vi "Run.vi"(8 "error in (no error)":errorcluster, 11 "SiemensDigitalEnergyMeter in":refnum<class "SiemensDigitalEnergyMeter.lvclass">) -> (0 "error out":errorcluster, 1 "DataValid":bool, 2 "clSensorData":T1, 3 "SiemensDigitalEnergyMeter out":refnum<class "SiemensDigitalEnergyMeter.lvclass">)   [LabVIEW 2018, in "SensorPlugins.lvlib" / "SiemensDigitalEnergyMeter.lvclass"]
doc: "This VI retrieves measurements from the Siemens Digital Energy Meter."
uses:
  SiemensDigitalEnergyMeter.lvclass
  SensorShared/clSensorData.ctl
  SensorShared/SiemensDEMMeasurements.ctl
  <vilib>/NI/Modbus Library/API/Master/Modbus Master.lvclass
  SensorShared/SensorShared.lvlib
panel:
  out "Execution Time (ms)":u32
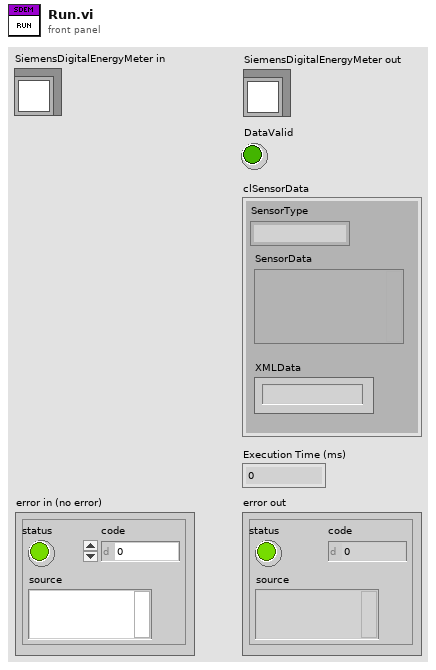
[diagram p1: front panel]
types:
  T1 = typedef "SensorShared.lvlib/clSensorData.ctl" = cluster{"SensorType":string, "SensorData":variant, "XMLData":string}
  T2 = typedef "SensorPlugins.lvlib/SiemensDigitalEnergyMeter.lvclass/CommunicationControls.ctl" = refnum<class "Modbus Master.lvclass">[]
  T3 = typedef "SensorPlugins.lvlib/SiemensDigitalEnergyMeter.lvclass/SiemensDigitalEnergyMeterControls.ctl" = cluster{"Measurement(s)":u16[], "Configuration Commands":string, "Use Measurement Commands Text Box?":bool, "Measurement Commands":string, "Connected?":bool, "Serial Number":string, "IP Address":string, "Port (502)":u16, "Unit ID":u8, "Serial Type":enum16{"RTU", "ASCII"}, "Using TCP?":bool, "VISA Resource Name":string}[]
  T4 = typedef "SensorPlugins.lvlib/SiemensDigitalEnergyMeter.lvclass/MeasurementControls.ctl" = cluster{"Measurement RefreshTime (ms)":u32, "Measurement Name":string}
  T5 = typedef "SensorShared.lvlib/SiemensDEMMeasurements.ctl" = cluster{"Array of Waveforms":waveform(dbl)[], "Array of Strings ":string[]}
  T6 = cluster{"Measurement(s)":u16[], "Configuration Commands":string, "Use Measurement Commands Text Box?":bool, "Measurement Commands":string, "Connected?":bool, "Serial Number":string, "IP Address":string, "Port (502)":u16, "Unit ID":u8, "Serial Type":enum16{"RTU", "ASCII"}, "Using TCP?":bool, "VISA Resource Name":string}
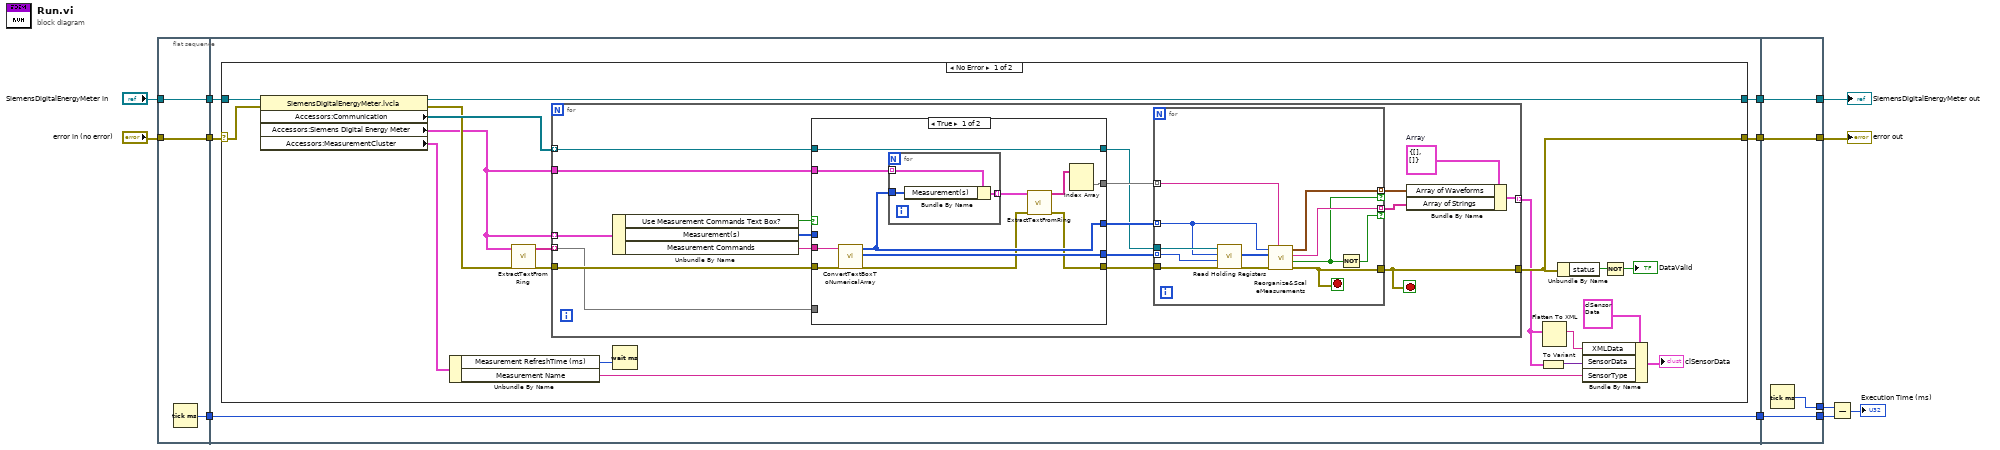
[diagram p0: block diagram]
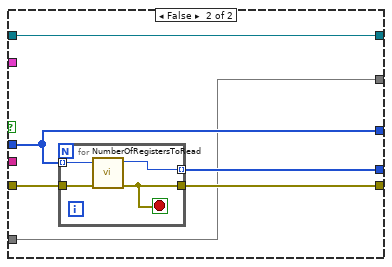
[diagram p2: hidden frame]
diagram:
  n1 = flat-sequence {
    tunnel: "SiemensDigitalEnergyMeter in" -> [w15]
    tunnel: "error in (no error)" -> [w16]
    tunnel: [w16] -> w9
    tunnel: [w15] -> w8
    tunnel: [w14] -> w7
    tunnel: w9 -> [w21]
    tunnel: w8 -> [w20]
    tunnel: [w19] -> w6
    tunnel: [w18] -> w5
    tunnel: w7 -> [w17]
    tunnel: [w17] -> w4
    tunnel: [w99] -> w10
    tunnel: [w100] -> w11
    tunnel: w4 -> [w97]
    tunnel: w5 -> [w99]
    tunnel: w6 -> [w100]
    tunnel: [w98] -> w2
    tunnel: [w97] -> w1
    frame #0 {
      n2 = Tick Count (ms)() -> (millisecond timer value=w14:u32)
    }
    frame #1 {
      n3 = case shown="No Error" w21 {
        selector: w21 -> [w39 w96]
        tunnel: w20 -> [w40 w95]
        tunnel: [w27 w96] -> w18
        tunnel: [w38 w95] -> w19
        frame No Error {
          n4 = property class="SiemensDigitalEnergyMeter.lvcla"(reference=w40, error in=w39) -> (reference out=w38:refnum<class "SiemensDigitalEnergyMeter.lvclass">, error out=w33:errorcluster, "Accessors:Communication"=w37:T2, "Accessors:Siemens Digital Energy Meter"=w30:T3, "Accessors:MeasurementCluster"=w26:T4)
          n5 = Unbundle By Name(w26) -> ("Measurement RefreshTime (ms)"=w25:u32, "Measurement Name"=w24:string)
          n6 = call "ExtractTextFromRing.vi"("error in (no error)"=w33, "Siemens Digital Energy Meter"=w30) -> ("error out"=w32:errorcluster, "MeasurementTypeStrings"=w31:string[][])  [unwired: 8 in]
          n7 = for {
            tunnel: w30 -> [w50] mode=indexing
            tunnel: w32 -> [w55]
            tunnel: [w54] -> w27
            tunnel: w37 -> [w42] mode=indexing
            tunnel: w31 -> [w48] mode=indexing
            tunnel: w30 -> [w49]
            tunnel: [w43] -> w22 mode=indexing
            stop <- w54 stop-if-true
            w46 = T5 {"Array of Waveforms"=[], "Array of Strings "=[]}  # Array
            n8 = Unbundle By Name(w50) -> ("Use Measurement Commands Text Box?"=w58:bool, "Measurement(s)"=w57:u16[], "Measurement Commands"=w56:string)
            n9 = case shown="True" w58 {
              tunnel: [w60 w77] -> w51
              tunnel: w57 -> [_ w76]
              tunnel: w56 -> [w68 _]
              tunnel: w55 -> [w69 w78]
              tunnel: [w66 w76] -> w53
              tunnel: [w67 w75] -> w52
              tunnel: w49 -> [w65 _]
              tunnel: w48 -> [_ w74]
              tunnel: [w61 w74] -> w47
              tunnel: w42 -> [w59 w73]
              tunnel: [w59 w73] -> w41
              frame True {
                n10 = call "ConvertTextBoxToNumericalArray.vi"("Error In"=w69, "Configuration Commands"=w68) -> ("Error Out"=w63:errorcluster, "Register Value"=w67:u16[], "Register"=w66:u16[])  [unwired: 7 in]
                n11 = for {
                  tunnel: w66 -> [w72]
                  tunnel: w65 -> [w71] mode=indexing
                  tunnel: [w70] -> w64 mode=indexing
                  n12 = Bundle By Name(cluster=w71, "Measurement(s)"=w72) -> (w70:T6)
                }
                n13 = call "ExtractTextFromRing.vi"("error in (no error)"=w63, "Siemens Digital Energy Meter"=w64) -> ("error out"=w60:errorcluster, "MeasurementTypeStrings"=w62:string[][])  [unwired: 8 in]
                n14 = Index Array(array=w62) -> (element=w61:string[])  [unwired: 2 in]
              }
              frame False {
                n15 = for {
                  tunnel: [w81] -> w75 mode=indexing
                  tunnel: w76 -> [w80] mode=indexing
                  tunnel: w78 -> [w82]
                  tunnel: [w79] -> w77
                  stop <- w79 stop-if-true
                  n16 = call "NumberOfRegistersToRead.vi"("Error In"=w82, "Measurement TextRing"=w80) -> ("Error Out"=w79:errorcluster, "Numer of Registers"=w81:u16)  [unwired: 8 in]
                }
              }
            }
            n17 = for {
              tunnel: [w94] -> w54
              tunnel: [w93] -> w44 mode=indexing if=w90
              tunnel: [w92] -> w45 mode=indexing if=w91
              tunnel: w51 -> [w86]
              tunnel: w41 -> [w85]
              tunnel: w53 -> [w84] mode=indexing
              tunnel: w52 -> [w83] mode=indexing
              tunnel: w47 -> [w89] mode=indexing
              stop <- w94 stop-if-true
              n18 = call-dynamic "Read Holding Registers.vi"("error in"=w86, "number of inputs"=w83, "starting address"=w84, "Modbus master in"=w85) -> ("error out"=w88:errorcluster, "register values"=w87:u16[])  [unwired: 5 in, 1 out]
              n19 = call "Reorganize&ScaleMeasurements.vi"("MeasurementType"=w89, "Error In"=w88, "Register Values"=w87, "Measurement TextRing"=w84) -> ("Error Out"=w94:errorcluster, "Numerical Information"=w90:bool, "String"=w92:string, "output waveform"=w93:waveform(dbl))  [unwired: 4 in]
              n20 = Not(x=w90) -> (.not. x?=w91:bool)
            }
            n21 = Bundle By Name(cluster=w46, "Array of Waveforms"=w44, "Array of Strings"=w45) -> (w43:T5)
          }
          n22 = Wait (ms)(milliseconds to wait=w25) -> ()  [unwired: 1 out]
          n23 = To Variant(anything=w22) -> (Variant=w34:variant)
          n24 = Flatten To XML(anything=w22) -> (xml string=w23:string)
          n25 = Unbundle By Name(w27) -> ("status"=w28:bool)
          n26 = Bundle By Name(cluster=T1 {"SensorType"="", "SensorData"=variant, "XMLData"=""} ("clSensorData"), "XMLData"=w23, "SensorData"=w34, "SensorType"=w24) -> (→"clSensorData":T1)
          n27 = Not(x=w28) -> (.not. x?=→"DataValid":bool)
        }
        frame Error {
        }
      }
    }
    frame #2 {
      n28 = Tick Count (ms)() -> (millisecond timer value=w98:u32)
    }
  }
  n29 = Subtract(x=w2, y=w1) -> (x-y=→"Execution Time (ms)":u32)
  "error out" <- w10
  "SiemensDigitalEnergyMeter out" <- w11
